vi "SPD.No Pulses Test.vi"(8 "Error In":errorcluster, 11 "SPD.Stand Ctrl in":T1={"spdDeviceSession"={"spdRef"=0, "connected"=FALSE, "spdName"="", "specification"={"diod case"=enum."default", "type"=enum."Unknown", "frequency"=enum."Unknown"}, "hidSPD.Controller"={"TSet"=0.0, "HV_bias"=0.0, "DDS_stb_code"=0}, "hidSPD.Sturtup Values"={"TSet"=0.0, "HV_bias"=0.0, "DDS_stb_code"=0}}, "DevBSession"={"DevBRef"="", "connected"=FALSE}, "FreqCSession"={"FreqCRef"="", "timeout"=0.0, "Gate"=0.0, "connected"=FALSE}, "8164BSession"={"Connection ID"=refnum, "Connected"=FALSE, "Info"="", "Slots Info"=[]}, "LeCroySession"={"LeCroySession"="", "connected"=FALSE}, "Events"={"DCRTest"=refnum, "Stop"=refnum}, "configFile"={"configFile ref"=refnum, "configFile path"=path "", "equipmentFile ref"=refnum}, "SPD.Meas Grid"={"DateTime"="", "DT"=[], "Insensitivity"=[], "Temprature"=[], "Stb_code"=[], "HV_Bias"=[]}, "SPD.Queues"={"state queue"=refnum}, "Console"=refnum} {"spdDeviceSession"."hidSPD.Sturtup Values"."HV_bias" format="%#_6p, V"; "spdDeviceSession"."hidSPD.Sturtup Values"."TSet" format="%#_6p, DegC"; "spdDeviceSession"."hidSPD.Controller"."HV_bias" format="%#_6p, V"; "spdDeviceSession"."hidSPD.Controller"."TSet" format="%#_6p, DegC"}) -> (0 "Error Out":errorcluster, 1 "pass":bool, 3 "SPD.Stand Ctrl out":T1={"spdDeviceSession"={"spdRef"=0, "connected"=FALSE, "spdName"="", "specification"={"diod case"=enum."default", "type"=enum."Unknown", "frequency"=enum."Unknown"}, "hidSPD.Controller"={"TSet"=0.0, "HV_bias"=0.0, "DDS_stb_code"=0}, "hidSPD.Sturtup Values"={"TSet"=0.0, "HV_bias"=0.0, "DDS_stb_code"=0}}, "DevBSession"={"DevBRef"="", "connected"=FALSE}, "FreqCSession"={"FreqCRef"="", "timeout"=0.0, "Gate"=0.0, "connected"=FALSE}, "8164BSession"={"Connection ID"=refnum, "Connected"=FALSE, "Info"="", "Slots Info"=[]}, "LeCroySession"={"LeCroySession"="", "connected"=FALSE}, "Events"={"DCRTest"=refnum, "Stop"=refnum}, "configFile"={"configFile ref"=refnum, "configFile path"=path "", "equipmentFile ref"=refnum}, "SPD.Meas Grid"={"DateTime"="", "DT"=[], "Insensitivity"=[], "Temprature"=[], "Stb_code"=[], "HV_Bias"=[]}, "SPD.Queues"={"state queue"=refnum}, "Console"=refnum} {"spdDeviceSession"."hidSPD.Sturtup Values"."HV_bias" format="%#_6p, V"; "spdDeviceSession"."hidSPD.Sturtup Values"."TSet" format="%#_6p, DegC"; "spdDeviceSession"."hidSPD.Controller"."HV_bias" format="%#_6p, V"; "spdDeviceSession"."hidSPD.Controller"."TSet" format="%#_6p, DegC"})   [LabVIEW 2018]
uses:
  typedefs/SPD.Stand Ctrl.ctl
  Instruments/SPD HID Interface/hidSPDLibForLabView/LibVIs/hidSPD Controls/hidSPD Device Session.ctl
  Instruments/SPD HID Interface/hidSPDLibForLabView/LibVIs/hidSPD Controls/hidSPD.SPD specification.ctl
  Instruments/SPD HID Interface/hidSPDLibForLabView/LibVIs/hidSPD Controls/hidSPD SPD Diod Case.ctl
  Instruments/SPD HID Interface/hidSPDLibForLabView/LibVIs/hidSPD Controls/hidSPD SPD Type.ctl
  Instruments/SPD HID Interface/hidSPDLibForLabView/LibVIs/hidSPD Controls/hidSPD.STB Frequency.ctl
  Instruments/SPD HID Interface/hidSPDLibForLabView/LibVIs/hidSPD Controls/hidSPD Controller.ctl
  Instruments/KC705 DevBoard/typedefs/DevB.Session.ctl
  Instruments/KeySight 53230A/typedefs/FreqC.Session.ctl
  Instruments/KeySight 8164B/KeySight 8164B LAN InstrLib/typedefs/KeySight 8164B control.ctl
  Instruments/LeCroy SDA830/typedefs/LeCroy.Session.ctl
  typedefs/SPD.Events.ctl
  ConfigFile/SPD.Config File ctrl.ctl
  <vilib>/Utility/config.llb/Config Data RefNum.ctl
  typedefs/SPD.Meas Grid.ctl
  typedefs/SPD.Queues.ctl
  typedefs/SPD.Stand state.ctl
  Instruments/SPD HID Interface/hidSPDLibForLabView/LibVIs/hidSPD Controls/hidSPD Controller Setup Report.ctl
  Instruments/SPD HID Interface/hidSPDLibForLabView/LibVIs/hidSPD Write Report/hidSPD Setup Controller.vi
  Instruments/SPD HID Interface/hidSPDLibForLabView/hidSPDLibForLabView.lvlib
  Instruments/KeySight 8164B/KeySight 8164B LAN InstrLib.lvlib
  <vilib>/Utility/config.llb/NI_LVConfig.lvlib
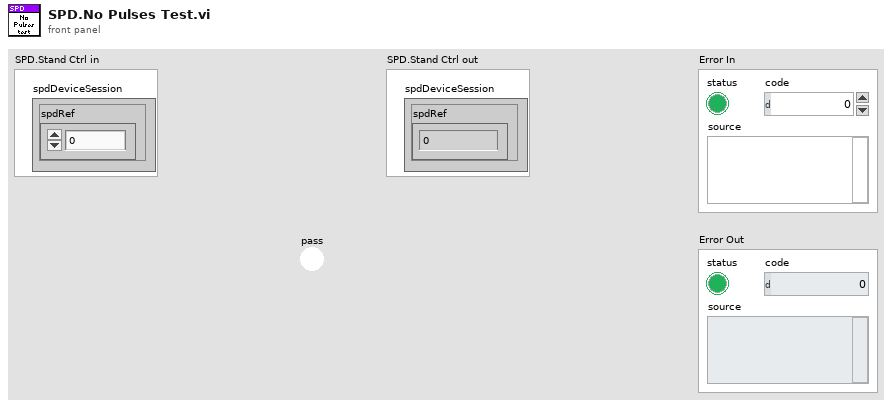
[diagram p1: front panel]
types:
  T1 = typedef "SPD.Stand Ctrl.ctl" = cluster{"spdDeviceSession":T2, "DevBSession":T8, "FreqCSession":T9, "8164BSession":T10, "LeCroySession":T11, "Events":T12, "configFile":T13, "SPD.Meas Grid":T15, "SPD.Queues":T16, "Console":refnum<vi>}
  T2 = typedef "hidSPDLibForLabView.lvlib/hidSPD Device Session.ctl" = cluster{"spdRef":u64, "connected":bool, "spdName":string, "specification":T3, "hidSPD.Controller":T7, "hidSPD.Sturtup Values":T7}
  T3 = typedef "hidSPDLibForLabView.lvlib/hidSPD.SPD specification.ctl" = cluster{"diod case":T4, "type":T5, "frequency":T6}
  T4 = typedef "hidSPDLibForLabView.lvlib/hidSPD SPD Diod Case.ctl" = enum16{"Unknown", "default", "butterfly"}
  T5 = typedef "hidSPDLibForLabView.lvlib/hidSPD SPD Type.ctl" = enum16{"Unknown", "Free Run", "Gate"}
  T6 = typedef "hidSPDLibForLabView.lvlib/hidSPD.STB Frequency.ctl" = enum16{"Unknown", "312", "1250"}
  T7 = typedef "hidSPDLibForLabView.lvlib/hidSPD Controller.ctl" = cluster{"TSet":sgl, "HV_bias":sgl, "DDS_stb_code":u16}
  T8 = typedef "DevB.Session.ctl" = cluster{"DevBRef":refnum<visa-resource-name>, "connected":bool}
  T9 = typedef "FreqC.Session.ctl" = cluster{"FreqCRef":refnum<visa-resource-name>, "timeout":dbl, "Gate":dbl, "connected":bool}
  T10 = typedef "KeySight 8164B LAN InstrLib.lvlib/KeySight 8164B control.ctl" = cluster{"Connection ID":refnum<k5>, "Connected":bool, "Info":string, "Slots Info":string[]}
  T11 = typedef "LeCroy.Session.ctl" = cluster{"LeCroySession":refnum<visa-resource-name>, "connected":bool}
  T12 = typedef "SPD.Events.ctl" = cluster{"DCRTest":refnum<user-event>, "Stop":refnum<user-event>}
  T13 = typedef "SPD.Config File ctrl.ctl" = cluster{"configFile ref":T14, "configFile path":path, "equipmentFile ref":T14}
  T14 = typedef "NI_LVConfig.lvlib/Config Data RefNum.ctl" = refnum<k1>
  T15 = typedef "SPD.Meas Grid.ctl" = cluster{"DateTime":string, "DT":dbl[], "Insensitivity":dbl[], "Temprature":dbl[], "Stb_code":dbl[], "HV_Bias":dbl[][][][]}
  T16 = typedef "SPD.Queues.ctl" = cluster{"state queue":refnum<queue>}
  T17 = typedef "hidSPDLibForLabView.lvlib/hidSPD Controller Setup Report.ctl" = cluster{"TSet":sgl, "HV_bias":sgl, "DDS_stb_code":u16, "SPD_reset":u16, "MCU_reset":u16}
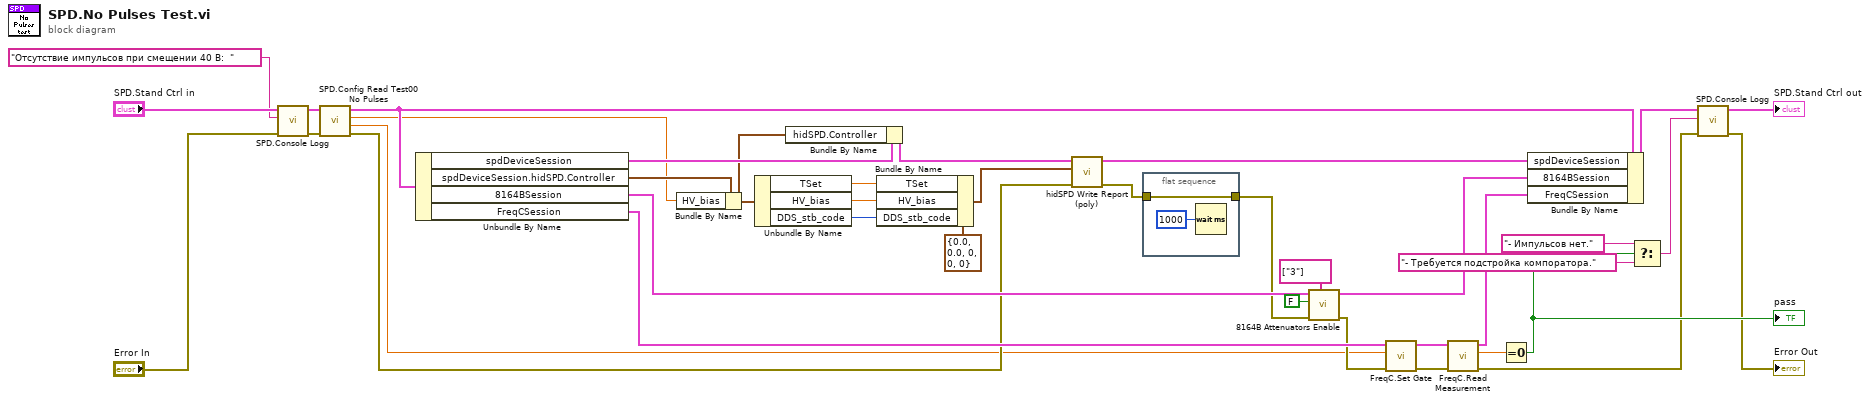
[diagram p0: block diagram]
diagram:
  n1 = call "SPD.Console Logg.vi"("Error In"="Error In", "console Log"="Отсутствие импульсов при смещении 40 В:  ", "SPD.Stand Ctrl in"="SPD.Stand Ctrl in") -> ("Error Out"=w8:errorcluster, "SPD.Stand Ctrl out"=w9:T1)  [unwired: 7 in]
  n2 = call "SPD.Config Read Test00 No Pulses.vi"("Error In"=w8, "SPD.Stand Ctrl in"=w9) -> ("Error Out"=w15:errorcluster, "FreqC_GateTime"=w13:dbl, "HV_bias"=w14:dbl, "SPD.Stand Ctrl out"=w16:T1)  [unwired: 6 in]
  n3 = Unbundle By Name(w16) -> ("spdDeviceSession"=w39:T2, "spdDeviceSession.hidSPD.Controller"=w37:T7, "8164BSession"=w32:T10, "FreqCSession"=w30:T9)
  n4 = Bundle By Name(cluster=w37, "HV_bias"=w14) -> (w24:T7)
  n5 = Unbundle By Name(w24) -> ("TSet"=w36:sgl, "HV_bias"=w35:sgl, "DDS_stb_code"=w34:u16)
  n6 = Bundle By Name(cluster=w39, "hidSPD.Controller"=w24) -> (w25:T2)
  n7 = Bundle By Name(cluster=T17 {"TSet"=0.0, "HV_bias"=0.0, "DDS_stb_code"=0, "SPD_reset"=0, "MCU_reset"=0} ("hidSPD Controller Setup report"), "TSet"=w36, "HV_bias"=w35, "DDS_stb_code"=w34) -> (w33:T17)
  n8 = call-poly "hidSPD Write Report (poly).vi"("error in (no error)"=w15, "hidSPD Controller Setup report"=w33, "spdDevSession in"=w25) -> ("error out"=w12:errorcluster, "spdDevSession out"=w26:T2)  [unwired: 7 in]
  n9 = flat-sequence {
    tunnel: w12 -> [w41]
    tunnel: [w41] -> w11
    frame #0 {
      n10 = Wait (ms)(milliseconds to wait=u32 1000) -> ()  [unwired: 1 out]
    }
  }
  n11 = call "8164B Attenuators Enable.vi"("Slots"=string[] ["3"], "error in"=w11, "Enable"=FALSE, "KeySight 8164B control in"=w32) -> ("error out"=w29:errorcluster, "KeySight 8164B control out"=w23:T10)  [unwired: 6 in]
  n12 = call "FreqC.Set Gate.vi"("error In"=w29, "Gate, sec"=w13, "FreqC Session in"=w30) -> ("error out"=w28:errorcluster, "FreqC Session out"=w27:T9)  [unwired: 7 in]
  n13 = call "FreqC.Read Measurement.vi"("error In"=w28, "FreqC Session in"=w27) -> ("error out"=w2:errorcluster, "Measurement"=w21:dbl, "FreqC Session out"=w22:T9)  [unwired: 7 in]
  n14 = Equal To 0?(x=w21) -> (x = 0?=w19:bool)
  "pass" <- w19
  n15 = Bundle By Name(cluster=w16, "spdDeviceSession"=w26, "8164BSession"=w23, "FreqCSession"=w22) -> (w5:T1)
  n16 = Select(t="- Импульсов нет." ("report"), s=w19, f="- Требуется подстройка компоратора.") -> (s? t:f=w3:string)
  n17 = call "SPD.Console Logg.vi"("Error In"=w2, "console Log"=w3, "SPD.Stand Ctrl in"=w5) -> ("Error Out"=→"Error Out":errorcluster, "SPD.Stand Ctrl out"=→"SPD.Stand Ctrl out":T1)  [unwired: 7 in]
